vi "golpi_mpc_command.vi"(5 "clear function cache before command? (False)":bool, 7 "timeout [ms]":u32=10000, 8 "error in":errorcluster, 10 "command":string, 11 "GOLPI ref in":T1={"pipe handle"={"lv_proc.dll file path"=path "", "process instance handle"=[], "debug mode"=FALSE, "debug data"=[]}, "fast read timeout [ms]"=500, "fast read settle time [ms]"=10, "fast read to multiple [ms]"=1, "max elements per input line"=100, "slow read timeout [ms]"=5000, "stdin double format specifier"="%_16e", "max elements per stdout output column"=100, "console mode bitstream"=FALSE, "bitstream first read timeout [ms]"=1000, "bitstream read timeout [ms]"=50, "struct transfer possible"=FALSE}) -> (0 "error out":errorcluster, 2 "read buffer":string, 3 "GOLPI ref. out":T1={"pipe handle"={"lv_proc.dll file path"=path "", "process instance handle"=[], "debug mode"=FALSE, "debug data"=[]}, "fast read timeout [ms]"=500, "fast read settle time [ms]"=10, "fast read to multiple [ms]"=1, "max elements per input line"=100, "slow read timeout [ms]"=5000, "stdin double format specifier"="%_16e", "max elements per stdout output column"=100, "console mode bitstream"=FALSE, "bitstream first read timeout [ms]"=1000, "bitstream read timeout [ms]"=50, "struct transfer possible"=FALSE})   [LabVIEW 2013, in "GOLPI Multi Process.lvlib"]
doc: "Multi-process GOLPI command. Call this when you need to execute GOLPI command (equivalent of GOLPI write) but it will also wait for command execution for a given timeout. Then it will return command text output.\nOptionally it will prepend function cache clear command. This is useful for debug because sometimes Octave does not update called functions even if they changed on the disk."
uses:
  GOLPI Multi Process.lvlib
  GOLPI Library.lvlibp/Public/GOLPI reference Type Def.ctl
  GOLPI Library.lvlibp/LV Process source distribution/Pipe Handle.ctl
  GOLPI Library.lvlibp
  GOLPI Library.lvlibp/LV Process source distribution/LV Process library.lvlib
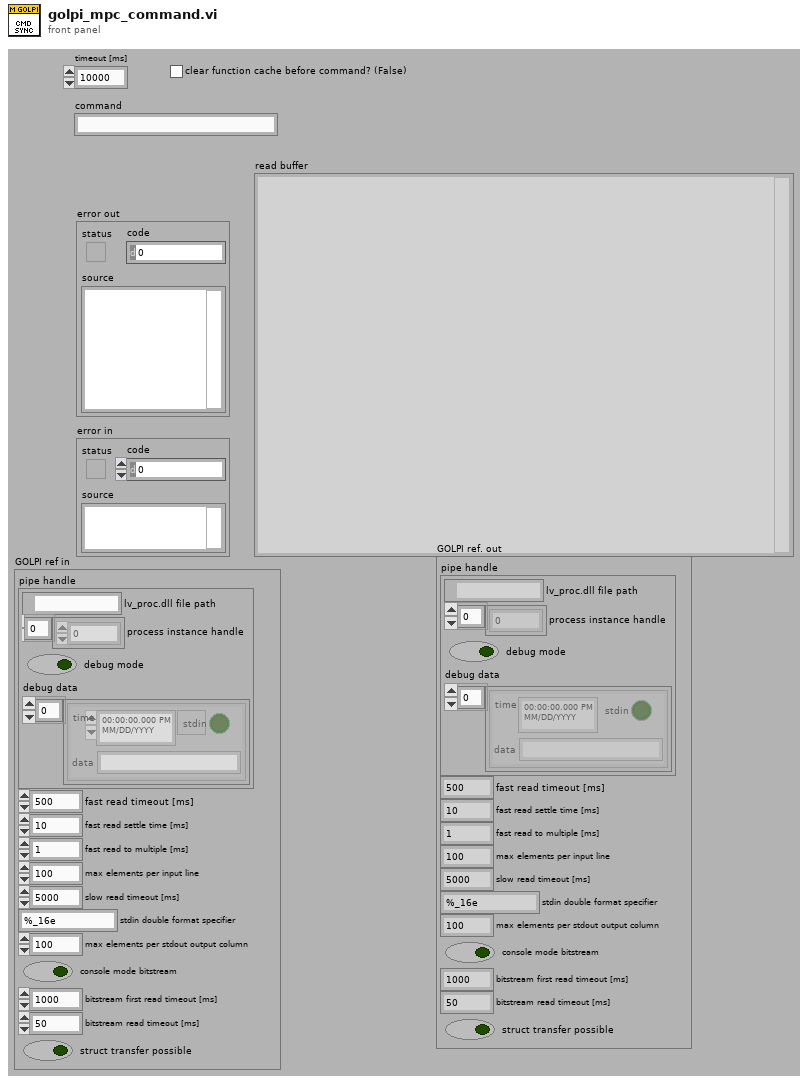
[diagram p1: front panel]
types:
  T1 = typedef "GOLPI Library.lvlibp/GOLPI reference Type Def.ctl" = cluster{"pipe handle":T2, "fast read timeout [ms]":u32, "fast read settle time [ms]":u32, "fast read to multiple [ms]":u32, "max elements per input line":u32, "slow read timeout [ms]":u32, "stdin double format specifier":string, "max elements per stdout output column":u32, "console mode bitstream":bool, "bitstream first read timeout [ms]":u32, "bitstream read timeout [ms]":u32, "struct transfer possible":bool}
  T2 = typedef "GOLPI Library.lvlibp/LV Process library.lvlib/Pipe Handle.ctl" = cluster{"lv_proc.dll file path":path, "process instance handle":u32[], "debug mode":bool, "debug data":cluster{"time":timestamp, "stdin":bool, "data":string}[]}
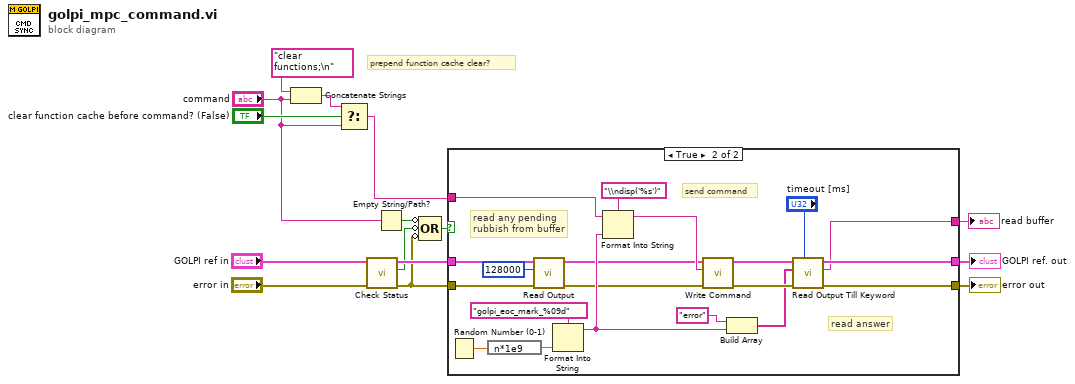
[diagram p0: block diagram]
diagram:
  # "prepend function cache clear?"
  n1 = Concatenate Strings("clear functions;\n" ("string"), "command") -> (w4:string)
  n2 = Select(t=w4, s="clear function cache before command? (False)", f="command") -> (s? t:f=w5:string)
  n3 = call "Check Status.vi"("error in"="error in", "GOLPI ref. in"="GOLPI ref in") -> ("error out"=w7:errorcluster, "exited?"=w8:bool, "GOLPI ref. out"=w12:T1)  [unwired: 7 in]
  n4 = Empty String/Path?(string/path="command") -> (empty?=w9:bool)
  n5 = Compound Arithmetic op=OR(invert w9, invert w8, invert w7) -> (w10:bool)
  n6 = case shown="True" w10 {
    tunnel: w7 -> [w17 w23]
    tunnel: w12 -> [w16 w22]
    tunnel: [w17 w34] -> w15
    tunnel: [w16 w33] -> w14
    tunnel: w5 -> [_ w27]
    tunnel: [_ w18] -> w1
    frame False {
    }
    frame True {
      # "read answer"
      # "send command"
      # "read any pending\nrubbish from buffer"
      n7 = Random Number (0-1)() -> (number: 0 to 1=w31:dbl)
      n8 = expression code="n*1e9"(w31) -> (w30:dbl)
      n9 = call "Read Output.vi"("error in"=w23, "byte count"=128000, "GOLPI ref. in"=w22) -> ("error out"=w20:errorcluster, "GOLPI ref. out"=w21:T1)  [unwired: 5 in, 2 out]
      n10 = Format Into String(format string="golpi_eoc_mark_%09d", w30) -> (resulting string=w25:string)  [unwired: 2 in, 1 out]
      n11 = Format Into String(format string="\\ndisp('%s')", initial string=w27, w25) -> (resulting string=w24:string)  [unwired: 1 in, 1 out]
      n12 = call "Write Command.vi"("error in"=w20, "command"=w24, "GOLPI ref. in"=w21) -> ("error out"=w37:errorcluster, "GOLPI ref. out"=w36:T1)  [unwired: 7 in]
      n13 = Build Array("error" ("keyword"), w25) -> (w29:string[])
      n14 = call "Read Output Till Keyword.vi"("timeout [ms]"="timeout [ms]", "error in"=w37, "keywords"=w29, "GOLPI ref. in"=w36) -> ("error out"=w34:errorcluster, "read buffer"=w18:string, "GOLPI ref. out"=w33:T1)  [unwired: 4 in, 1 out]
    }
  }
  "error out" <- w15
  "GOLPI ref. out" <- w14
  "read buffer" <- w1
